vi "2019-05-08_03.vi"() -> ()   [LabVIEW 2018]
panel:
  out "추가된 배열 2":dbl[](array[numeric])
  out "추가된 배열":dbl[][](array[numeric])
  in  "원소":dbl[](array[numeric])
  in  "배열":dbl[][](array[numeric])
  out "원소의 인덱스":i32
  in  "클러스터":T1
  out "출력 클러스터":T2
  in  "성별":bool
  in  "나이":dbl
  in  "주소":string
  in  "이름":string
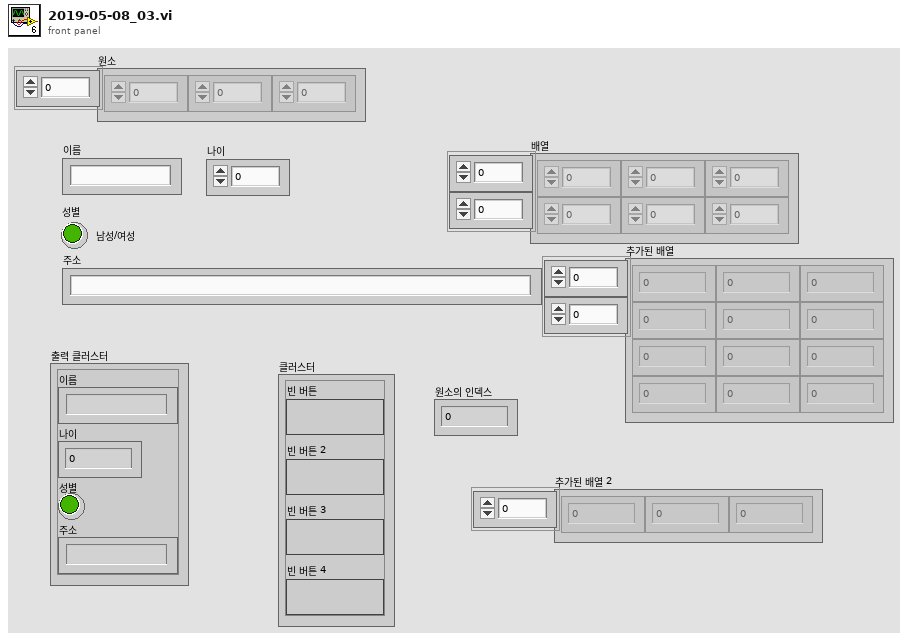
[diagram p1: front panel]
types:
  T1 = cluster{"빈 버튼":bool, "빈 버튼 2":bool, "빈 버튼 3":bool, "빈 버튼 4":bool}
  T2 = cluster{"이름":string, "나이":dbl, "성별":bool, "주소":string}
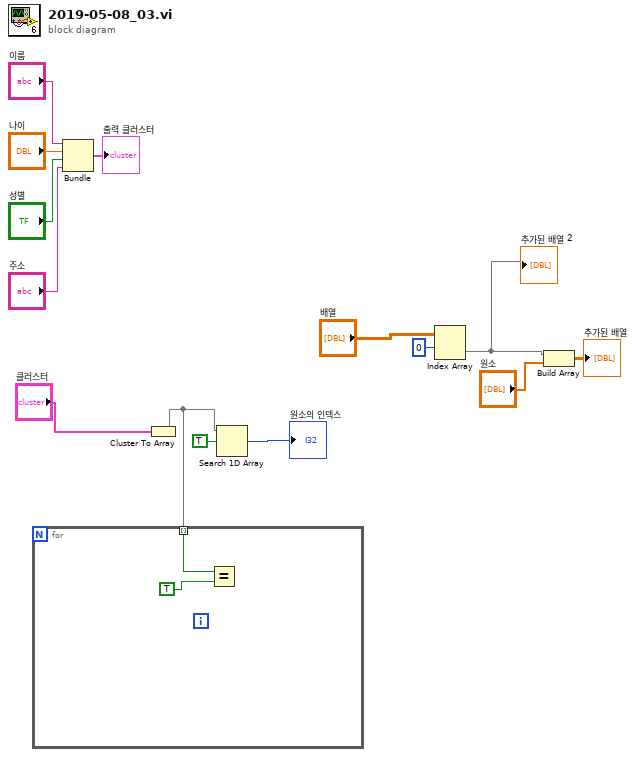
[diagram p0: block diagram]
diagram:
  n1 = Bundle("이름"="이름", "나이"="나이", "성별"="성별", "주소"="주소") -> (→"출력 클러스터":T2)  [unwired: 1 in]
  n2 = Cluster To Array(cluster="클러스터") -> (array=w1:bool[])
  n3 = for {
    tunnel: w1 -> [w16] mode=indexing
    n4 = Equal?(x=w16, y=TRUE) -> ()  [unwired: 1 out]
  }
  n5 = Search 1D Array(1D array=w1, element=TRUE ("원소")) -> (index of element=→"원소의 인덱스":i32)  [unwired: 1 in]
  n6 = Index Array(array="배열", index (row)=0 ("인덱스 (행)")) -> (element=w2:dbl[])  [unwired: 1 in]
  "추가된 배열 2" <- w2
  n7 = Build Array(w2, "원소") -> (→"추가된 배열":dbl[][])
